vi "Number of Results.vi"() -> (3 "number of results":i32=2)   [LabVIEW 2020, in "Light Test Case Double.lvclass"]
uses:
  Light Test Case Double.lvclass
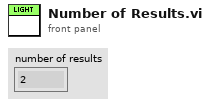
[diagram p1: front panel]
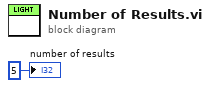
[diagram p0: block diagram]
diagram:
  "number of results" <- 5 ("y")
